vi "Motor.EvaluateStopCondition.vi"(6 "MotorBits":u8, 7 "Start Time":u32, 9 "StageDefinition":T2 {"Update Flags" format="%.0x"; "Goal Type" items=["Unlimited", "Distance", "Time", "Stop"]; "RunState" format="%02.0f" items=["IDLE"=0, "RAMPUP"=16, "RUNNING"=32, "RAMPDOWN"=64]; "RegMode" format="%02.0f" items=["IDLE", "SPEED", "SYNC"]; "Mode" format="%.0x"}, 10 "Wait?":bool, 11 "Motor":T6 items=["Port A", "Port B", "Port C"]) -> (2 "Canceled?":bool, 3 "Finished?":bool)   [LabVIEW 2009]
uses:
  <vilib>/NXT/Block Support/NXT_OutputPort.ctl
  MotorStageDefinition.ctl
  Move/RegMode.ctl
  Move/RunState.ctl
  <vilib>/NXT/Block Support/NXT_OutputGoalType.ctl
  NXTOutputRefnum.ctl
  Program Files/National Instruments/LabVIEW 2009/resource/objmgr/NXTInputOutput.rc
panel:
  in  "Generic Refnum Name":T1
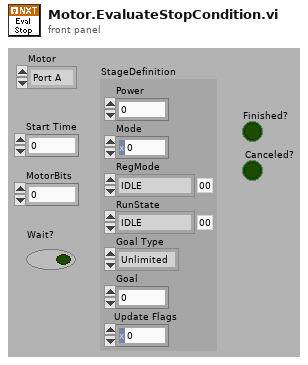
[diagram p1: front panel]
types:
  T1 = typedef "NXTOutputRefnum.ctl" = refnum<k21>
  T2 = typedef "MotorStageDefinition.ctl" = cluster{"Power":i8, "Mode":u8, "RegMode":T3, "RunState":T4, "Goal Type":T5, "Goal":u32, "Update Flags":u8}
  T3 = typedef "RegMode.ctl" = u8
  T4 = typedef "RunState.ctl" = u8
  T5 = typedef "NXT_OutputGoalType.ctl" = u16
  T6 = typedef "NXT_OutputPort.ctl" = u8
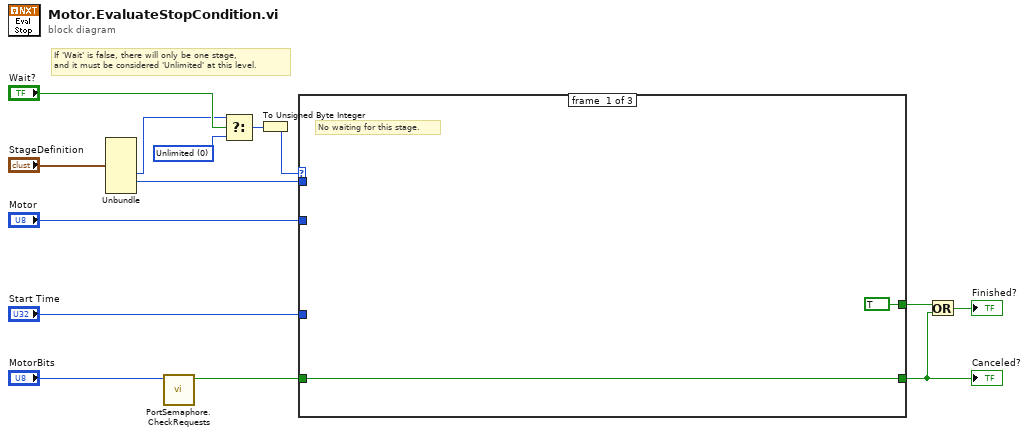
[diagram p0: block diagram]
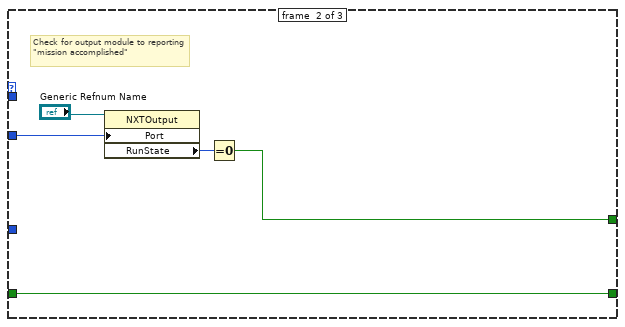
[diagram p2: hidden frame]
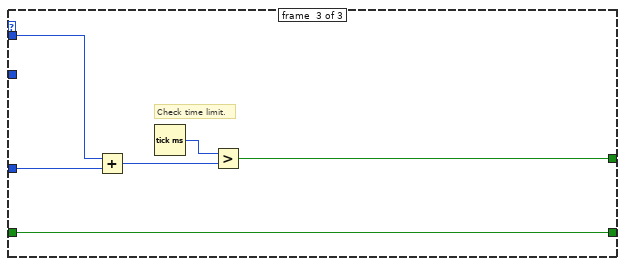
[diagram p3: hidden frame]
diagram:
  w5 = T5 0 items=["Unlimited", "Distance", "Time", "Stop"] ("f")
  # "If 'Wait' is false, there will only be one stage,\nand it must be considered 'Unlimited' at this level."
  n1 = Unbundle("StageDefinition") -> ("Goal Type"=w2:T5, "Goal"=w14:u32)  [unwired: 5 out]
  n2 = call <vilib>:"PortSemaphore.CheckRequests.vi"("MotorBits"="MotorBits") -> ("Request?"=w11:bool)  [unwired: 10 in]
  n3 = Select(t=w2, s="Wait?", f=w5) -> (s? t:f=w4:T5)
  n4 = To Unsigned Byte Integer(number=w4) -> (unsigned 8bit integer=w1:u8)
  n5 = case shown="1" w1 {
    tunnel: w14 -> [_ _ w27]
    tunnel: "Motor" -> [_ w17 _]
    tunnel: "Start Time" -> [_ _ w24]
    tunnel: w11 -> [w15 w21 w22]
    tunnel: [w15 w21 w22] -> w10
    tunnel: [TRUE w20 w23] -> w9
    frame #0 {
      # "No waiting for this stage."
    }
    frame #1 {
      # "Check for output module to reporting \"mission accomplished\""
      n6 = property class="NXTOutput"(reference="Generic Refnum Name", "Port"=w17) -> ("RunState"=w19:u8)  [unwired: 1 in, 2 out]
      n7 = Equal To 0?(x=w19) -> (x = 0?=w20:bool)
    }
    frame #2 {
      # "Check time limit."
      n8 = Add(x=w27, y=w24) -> (x+y=w26:u32)
      n9 = Tick Count (ms)() -> (millisecond timer value=w25:u32)
      n10 = Greater?(x=w25, y=w26) -> (0:w23:bool)
    }
  }
  "Canceled?" <- w10
  n11 = Or(x=w9, y=w10) -> (x .or. y?=→"Finished?":bool)
